vi "B_calibration_ramp.vi"() -> ()   [LabVIEW 2015]
doc: "Use this template to build a producer/consumer design pattern. Use this template when you need to execute a process, such as data analysis, when a data source, such as a triggered acquisition, produces data at an uneven rate and you need to execute the process when the data becomes available."
uses:
  oxford_driver/Oxford Drivers/BUSGEN.LLB/OxfordAddress.ctl
  <vilib>/Utility/file.llb/Write Delimited Spreadsheet (DBL).vi
panel:
  out "appended array":dbl[][](array[numeric])
  in  "Set Field (T)":dbl=0.3
  in  "stop":bool
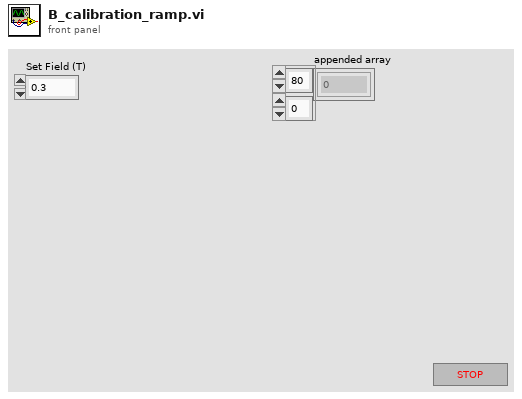
[diagram p1: front panel]
types:
  T1 = typedef "OxfordAddress.ctl" = cluster{"Com Port":i32, "ISOBUS Address":i32, "GPIB Address":i16, "Communication":enum16{"RS232", "ISOBUS", "GPIB", "Gateway"}}
  T2 = cluster{"read buffer":string, "Reply":string, "Reply":string}
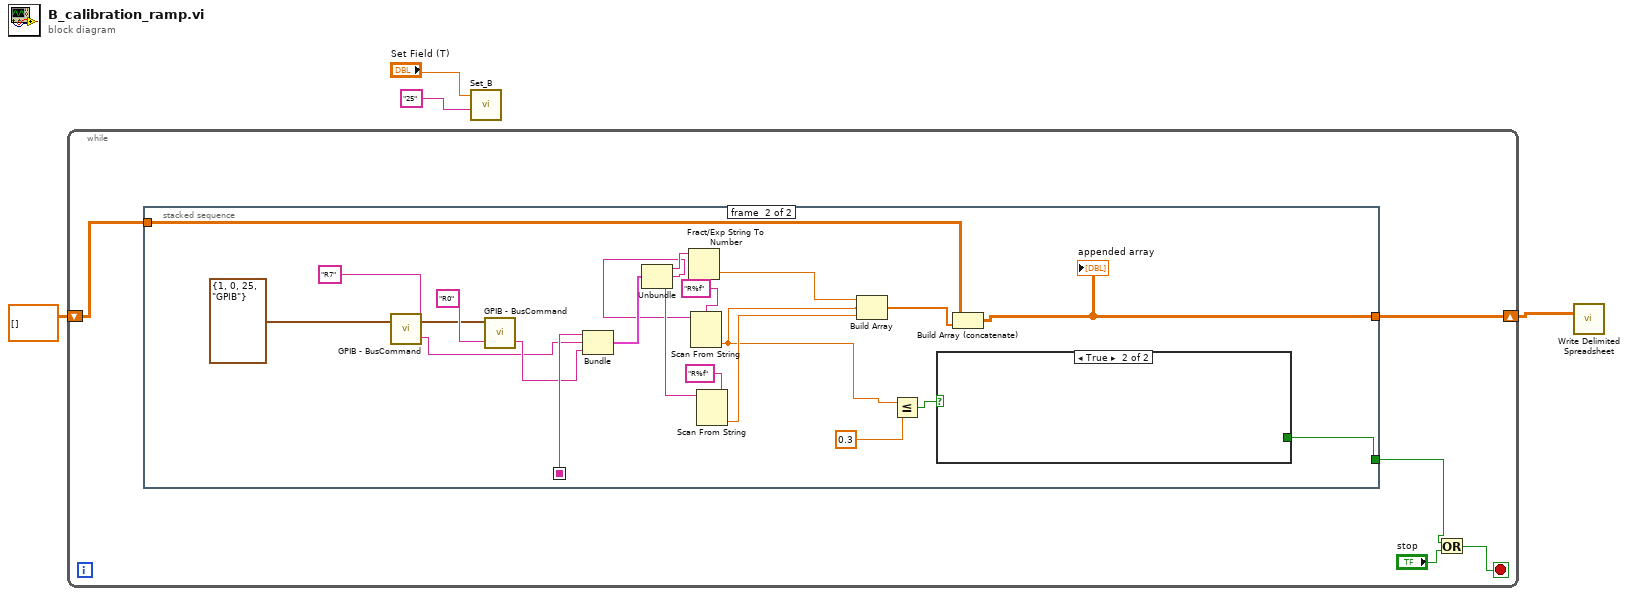
[diagram p0: block diagram]
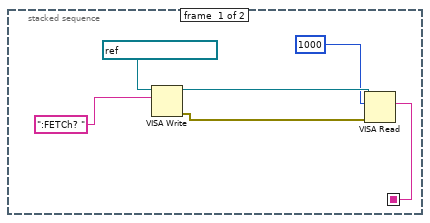
[diagram p2: hidden frame]
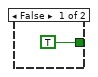
[diagram p3: hidden frame]
diagram:
  n1 = while {
    shift-right: [w9] -> w4
    shift-left: dbl[][] [] -> [w8]
    stop <- w5 stop-if-true
    n2 = stacked-sequence {
      seq-local: [w10 _] -> [_ w28]
      tunnel: [_ w23] -> w9
      tunnel: w8 -> [_ w22]
      tunnel: [_ w19] -> w7
      frame #0 {
        n3 = VISA Write(VISA resource name=refnum<visa-resource-name> "GPIB0::21::INSTR", write buffer=":FETCh? " ("data")) -> (VISA resource name out=w15:refnum<visa-resource-name>, error out=w11:errorcluster)  [unwired: 1 in, 1 out]
        n4 = VISA Read(VISA resource name=w15, byte count=u32 1000, error in (no error)=w11) -> (read buffer=w10:string)  [unwired: 3 out]
      }
      frame #1 {
        n5 = call "GPIB - BusCommand.vi"("Command"="R7" ("write buffer"), "Address"=T1 {"Com Port"=1, "ISOBUS Address"=0, "GPIB Address"=25, "Communication"=enum."GPIB"}) -> ("Reply"=w26:string, "Address(thru)"=w36:T1)
        n6 = call "GPIB - BusCommand.vi"("Command"="R0", "Address"=w36) -> ("Reply"=w27:string)  [unwired: 1 out]
        n7 = Bundle("read buffer"=w28, "Reply"=w26, "Reply"=w27) -> (w30:T2)  [unwired: 1 in]
        n8 = Unbundle(w30) -> ("read buffer"=w25:string, "Reply"=w17:string, "Reply"=w24:string)
        n9 = Fract/Exp String To Number(string=w25) -> (number=w32:dbl)  [unwired: 3 in, 1 out]
        n10 = Scan From String(format string="R%f" ("remaining string"), input string=w17) -> (output 1=w16:dbl)  [unwired: 3 in, 3 out]
        n11 = Scan From String(format string="R%f" ("remaining string"), input string=w24) -> (output 1=w33:dbl)  [unwired: 3 in, 3 out]
        n12 = Build Array(w32, w16, w33) -> (w31:dbl[])
        n13 = Less Or Equal?(x=w16, y=0.3) -> (x <= y?=w21:bool)
        n14 = case shown="True" w21 {
          tunnel: [TRUE _] -> w19
          frame False {
          }
          frame True {
          }
        }
        n15 = Build Array (concatenate)(w22, w31) -> (w23:dbl[][])
        "appended array" <- w23
      }
    }
    n16 = Or(x=w7, y="stop") -> (x .or. y?=w5:bool)
  }
  n17 = call "Set_B.vi"("address string"="25", "Set Field (T)"="Set Field (T)") -> ()  [unwired: 9 in, 1 out]
  n18 = call-poly <vilib>:"Write Delimited Spreadsheet.vi"("2D data"=w4) -> ()  [unwired: 13 in, 2 out]
